vi "Cancel State Machine - Load.vi"   [LabVIEW 2013]
uses:
  typedefs/State Machine/subStates.ctl
  typedefs/DevRef Type.ctl
  typedefs/fg_typedef.ctl
  typedefs/State Machine/singleUseSubstate.ctl
  <vilib>/Rock Robotics/WPI/Solenoid/WPI_SolenoidValue.ctl
  <vilib>/Rock Robotics/WPI/Solenoid/WPI_SolenoidGetEnum.vi
panel:
  # "A State Machine to Handle Canceling Load"
types:
  T1 = typedef "subStates.ctl" = enum16{"null", "wait", "driver control", "auto", "manual override", "hold position", "rotate", "pickup", "pass", "load", "goto shoot", "shoot high goal", "shoot low goal", "cancel arm", "cancel shooter", "end", "test"}
  T2 = typedef "fg_typedef.ctl" = enum16{"Get", "Set"}
  T3 = typedef "DevRef Type.ctl" = enum16{"Shooter Solenoid", "Latch Solenoid", "Right Up Sensor", "Right Down Sensor", "Hold Sensor", "2 Ball Switch", "Arm Encoder"}
  T4 = typedef "WPI_SolenoidValue.ctl" = enum16{"Off", "On", "Forward", "Reverse"}
  T5 = typedef "singleUseSubstate.ctl" = enum16{"null", "wait", "shift high", "shift low", "extend shooter", "retract shooter", "latch", "unlatch", "end"}
  T6 = typedef "WPI_DigitalInputDevRef.ctl" = cluster{"DevStatus":errorcluster, "DIO Channel":T7, "Digital Module":T8}
  T7 = typedef "FPGA_DIOChannel.ctl" = enum8{"DIO 1", "DIO 2", "DIO 3", "DIO 4", "DIO 5", "DIO 6", "DIO 7", "DIO 8", "DIO 9", "DIO 10", "DIO 11", "DIO 12", "DIO 13", "DIO 14", "Invalid"}
  T8 = typedef "FPGA_TypedefDigitalModule.ctl" = enum16{"Digital Module 1", "Digital Module 2"}
  T9 = typedef "WPI_SolenoidDevRef.ctl" = cluster{"DevStatus":errorcluster, "Solenoid Module":T10, "Forward Solenoid Channel":T11, "Reverse Solenoid Channel":T11}
  T10 = typedef "FPGA_TypedefSolenoidModule.ctl" = enum16{"Solenoid Module 1", "Solenoid Module 2"}
  T11 = typedef "WPI_SolenoidChannel.ctl" = enum8{"Solenoid 1", "Solenoid 2", "Solenoid 3", "Solenoid 4", "Solenoid 5", "Solenoid 6", "Solenoid 7", "Solenoid 8", "Invalid"}
  T12 = typedef "WPI_EncoderDevRef.ctl" = cluster{"DevStatus":errorcluster, "EncoderIndex":T13, "CounterIndex":T14, "DistancePerCount":dbl, "Decoding Type":T15}
  T13 = typedef "FPGA_EncoderIdx.ctl" = enum8{"Enc 0", "Enc 1", "Enc 2", "Enc 3", "Invalid"}
  T14 = typedef "FPGA_CounterCtrSystemIndex.ctl" = enum8{"Ctr 0", "Ctr 1", "Ctr 2", "Ctr 3", "Ctr 4", "Ctr 5", "Ctr 6", "Ctr 7", "Invalid"}
  T15 = typedef "WPI_EncoderType.ctl" = enum16{"1x", "2x", "4x"}
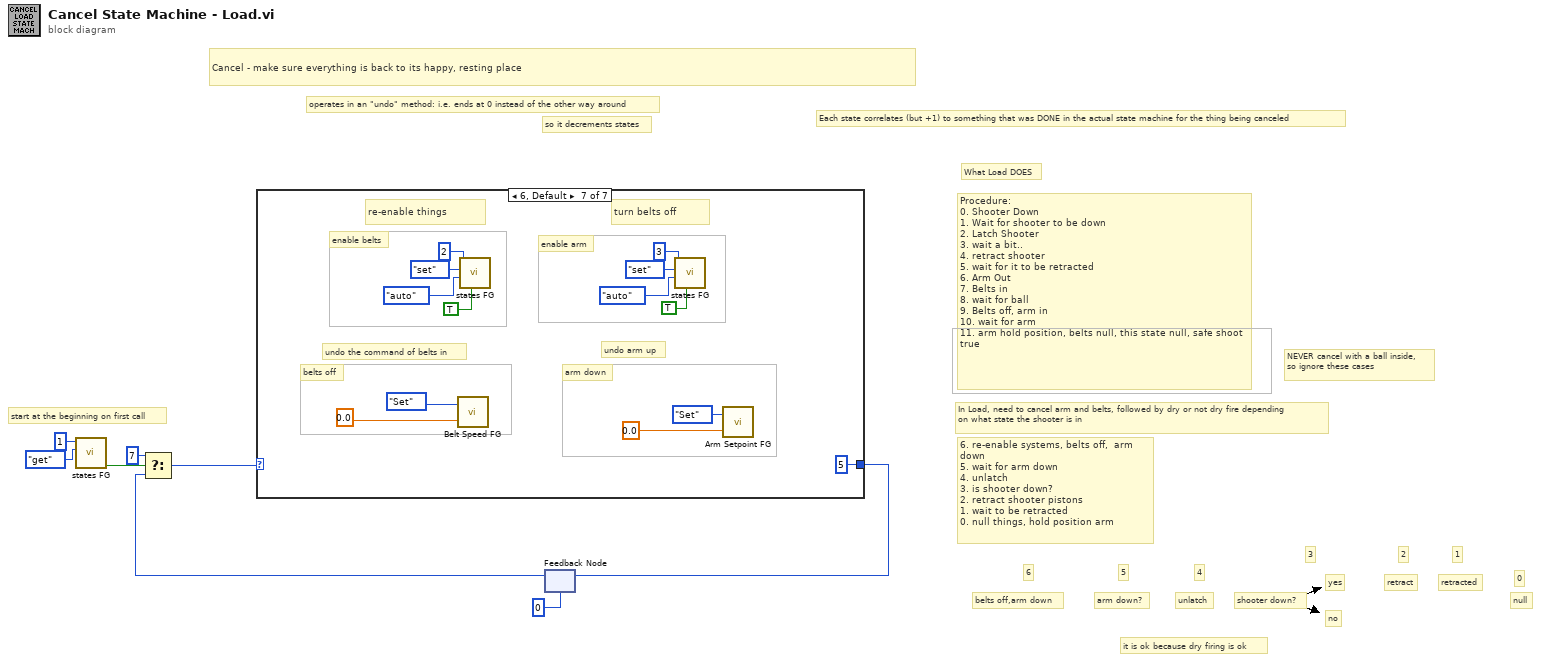
[diagram p0: block diagram]
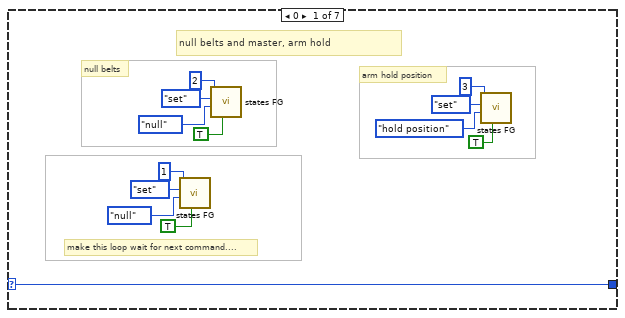
[diagram p2: hidden frame]
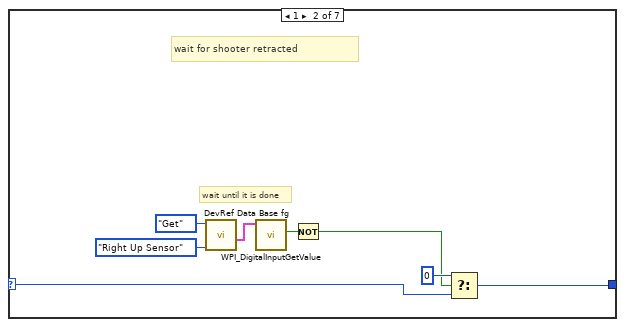
[diagram p3: hidden frame]
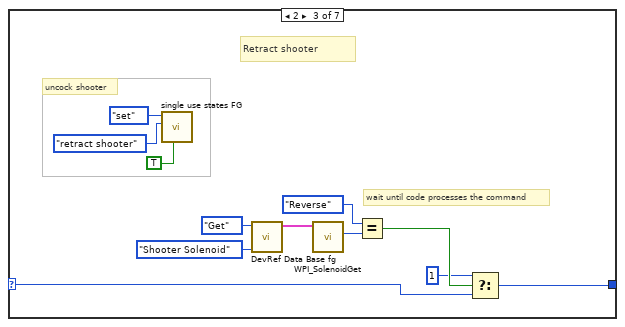
[diagram p4: hidden frame]
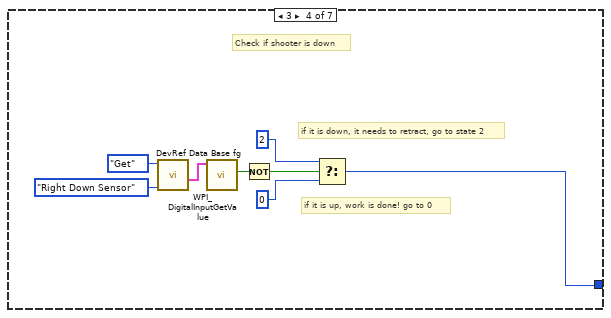
[diagram p5: hidden frame]
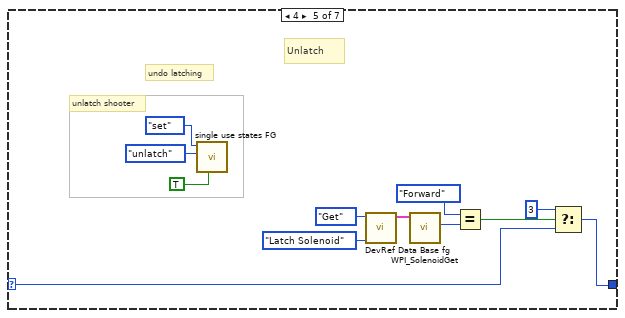
[diagram p6: hidden frame]
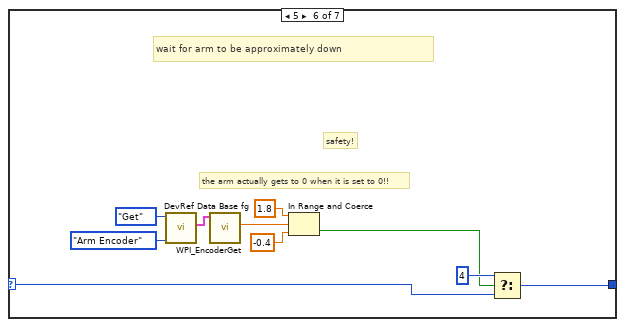
[diagram p7: hidden frame]
diagram:
  # "1"
  # "retracted"
  # "5"
  # "arm down?"
  # "it is ok because dry firing is ok"
  # "Procedure: \n0. Shooter Down \n1. Wait for shooter to be down\n2. Latch Shooter\n3. wait a bit..\n4. retract shooter\n5. wait for it to be retracted\n6. Arm Out\n7. Belts in\n8. wait for ball\n9. Belts off, arm in\n10. wait for arm\n11. arm hold position, belts null, this state null, safe shoot true"
  # "0"
  # "2"
  # "3"
  # "4"
  # "6"
  # "null"
  # "unlatch"
  # "retract"
  # "no"
  # "yes"
  # "shooter down?"
  # "belts off,arm down"
  # "NEVER cancel with a ball inside,\nso ignore these cases"
  # "What Load DOES"
  # "so it decrements states"
  # "Each state correlates (but +1) to something that was DONE in the actual state machine for the thing being canceled"
  # "6. re-enable systems, belts off,  arm down\n5. wait for arm down\n4. unlatch\n3. is shooter down?\n2. retract shooter pistons\n1. wait to be retracted\n0. null things, hold position arm"
  # "In Load, need to cancel arm and belts, followed by dry or not dry fire depending\non what state the shooter is in"
  # "operates in an \"undo\" method: i.e. ends at 0 instead of the other way around"
  # "start at the beginning on first call"
  # "Cancel - make sure everything is back to its happy, resting place"
  n1 = call "states FG.vi"("menu (get)"=enum16{"set", "get"}."get", "Loop ID"=1) -> ("first call?"=w8:bool)  [unwired: 6 in, 3 out]
  n2 = feedback #1(u8 0) -> (w3:u8)
  n3 = Select(t=u8 7, s=w8, f=w3) -> (s? t:f=w5:u8)
  n4 = case shown="6, Default" w5 {
    selector: w5 -> [w21 w27 w38 _ w54 w67 _]
    tunnel: [w21 w26 w37 w46 w53 w66 u8 5 ("t")] -> w2
    frame 0 {
      # "null belts and master, arm hold"
      # "make this loop wait for next command...."
      # "arm hold position"
      # "null belts"
      n5 = call "states FG.vi"("exit in"=TRUE, "subState in"=subStates."null", "menu (get)"=enum16{"set", "get"}."set", "Loop ID"=1) -> ()  [unwired: 4 in, 4 out]
      n6 = call "states FG.vi"("exit in"=TRUE, "subState in"=subStates."null", "menu (get)"=enum16{"set", "get"}."set", "Loop ID"=2) -> ()  [unwired: 4 in, 4 out]
      n7 = call "states FG.vi"("exit in"=TRUE, "subState in"=subStates."hold position", "menu (get)"=enum16{"set", "get"}."set", "Loop ID"=3) -> ()  [unwired: 4 in, 4 out]
    }
    frame 1 {
      # "wait until it is done"
      # "wait for shooter retracted"
      n8 = call "DevRef Data Base fg.vi"("DevRef to Get"=DevRef_Type."Right Up Sensor", "Menu"=fg_typedef."Get") -> ("Selected Sensor"=w28:T6)  [unwired: 2 in, 5 out]
      n9 = call <vilib>:"WPI_DigitalInputGetValue.vi"("DigitalInputDevRef"=w28) -> ("Value"=w29:bool)  [unwired: 8 in, 2 out]
      n10 = Not(x=w29) -> (.not. x?=w24:bool)
      n11 = Select(t=u8 0, s=w24, f=w27) -> (s? t:f=w26:u8)
    }
    frame 2 {
      # "wait until code processes the command"
      # "uncock shooter"
      # "Retract shooter"
      n12 = call "single use states FG.vi"("exit in"=TRUE, "substate"=singleUseSubstate."retract shooter", "menu (get)"=enum16{"set", "get"}."set") -> ()  [unwired: 5 in, 4 out]
      n13 = call "DevRef Data Base fg.vi"("DevRef to Get"=DevRef_Type."Shooter Solenoid", "Menu"=fg_typedef."Get") -> ("Selected Solenoid"=w36:T9)  [unwired: 2 in, 5 out]
      n14 = call-poly <vilib>:"WPI_SolenoidGet.vi"("SolenoidDevRef"=w36) -> ("Value"=w35:T4)  [unwired: 8 in, 2 out]
      n15 = Equal?(x=WPI_SolenoidValue."Reverse", y=w35) -> (x = y?=w33:bool)
      n16 = Select(t=u8 1, s=w33, f=w38) -> (s? t:f=w37:u8)
    }
    frame 3 {
      # "if it is up, work is done! go to 0"
      # "if it is down, it needs to retract, go to state 2"
      # "Check if shooter is down"
      n17 = call "DevRef Data Base fg.vi"("DevRef to Get"=DevRef_Type."Right Down Sensor", "Menu"=fg_typedef."Get") -> ("Selected Sensor"=w48:T6)  [unwired: 2 in, 5 out]
      n18 = call <vilib>:"WPI_DigitalInputGetValue.vi"("DigitalInputDevRef"=w48) -> ("Value"=w49:bool)  [unwired: 8 in, 2 out]
      n19 = Not(x=w49) -> (.not. x?=w47:bool)
      n20 = Select(t=u8 2, s=w47, f=u8 0) -> (s? t:f=w46:u8)
    }
    frame 4 {
      # "unlatch shooter"
      # "undo latching"
      # "Unlatch"
      n21 = call "single use states FG.vi"("exit in"=TRUE, "substate"=singleUseSubstate."unlatch", "menu (get)"=enum16{"set", "get"}."set") -> ()  [unwired: 5 in, 4 out]
      n22 = call "DevRef Data Base fg.vi"("DevRef to Get"=DevRef_Type."Latch Solenoid", "Menu"=fg_typedef."Get") -> ("Selected Solenoid"=w58:T9)  [unwired: 2 in, 5 out]
      n23 = call-poly <vilib>:"WPI_SolenoidGet.vi"("SolenoidDevRef"=w58) -> ("Value"=w56:T4)  [unwired: 8 in, 2 out]
      n24 = Equal?(x=WPI_SolenoidValue."Forward" ("Value"), y=w56) -> (x = y?=w55:bool)
      n25 = Select(t=u8 3, s=w55, f=w54) -> (s? t:f=w53:u8)
    }
    frame 5 {
      # "safety!"
      # "wait for arm to be approximately down"
      # "the arm actually gets to 0 when it is set to 0!!"
      n26 = call "DevRef Data Base fg.vi"("DevRef to Get"=DevRef_Type."Arm Encoder", "Menu"=fg_typedef."Get") -> ("Selected Encoder"=w71:T12)  [unwired: 2 in, 5 out]
      n27 = call <vilib>:"WPI_EncoderGet.vi"("EncoderDevRef"=w71) -> ("Distance"=w70:dbl)  [unwired: 5 in, 5 out]
      n28 = In Range and Coerce(upper limit=1.8, x=w70, lower limit=-0.4 ("upper limit")) -> (In Range?=w64:bool)  [unwired: 1 out]
      n29 = Select(t=u8 4, s=w64, f=w67) -> (s? t:f=w66:u8)
    }
    frame 6, Default {
      # "undo arm up"
      # "arm down"
      # "re-enable things"
      # "turn belts off"
      # "undo the command of belts in"
      # "belts off"
      # "enable arm"
      # "enable belts"
      n30 = call "Belt Speed FG.vi"("Speed In"=0.0 ("Setpoint In"), "Menu"=fg_typedef."Set") -> ()  [unwired: 1 out]
      n31 = call "states FG.vi"("exit in"=TRUE, "subState in"=subStates."auto", "menu (get)"=enum16{"set", "get"}."set", "Loop ID"=2) -> ()  [unwired: 4 in, 4 out]
      n32 = call "states FG.vi"("exit in"=TRUE, "subState in"=subStates."auto", "menu (get)"=enum16{"set", "get"}."set", "Loop ID"=3) -> ()  [unwired: 4 in, 4 out]
      n33 = call "Arm Setpoint FG.vi"("Setpoint In"=0.0, "Menu"=fg_typedef."Set") -> ()  [unwired: 1 out]
    }
  }
  n34 = feedback-in #1(w2) -> ()
